vi "tearDown.vi"(8 "error in (no error)":errorcluster, 11 "reference in":refnum<class "Instrument Addon Scripting API Channels Unit Tests.lvclass">) -> (0 "error out":errorcluster, 3 "reference out":refnum<class "Instrument Addon Scripting API Channels Unit Tests.lvclass">)   [LabVIEW 2018, in "Instrument Addon Scripting API Channels Unit Tests.lvclass"]
doc: "tearDown runs after the test method has completed. Use this method to clean up any operations or references that were opened by setUp or the test method. Unit tests should be independent of other unit tests so this VI should ensure that the next test can run in a 'clean' test environment."
uses:
  Instrument Addon Scripting API Channels Unit Tests.lvclass
  Instrument Addon Scripting API Channels Unit Tests.lvclass/Instrument Addon Scripting API Channels Unit Tests.ctl
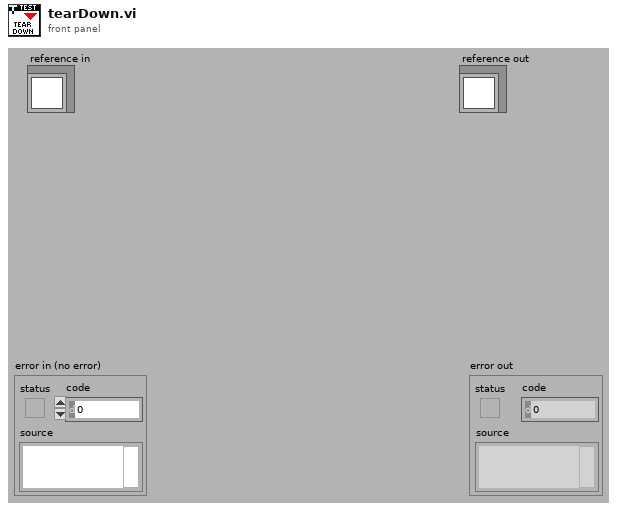
[diagram p1: front panel]
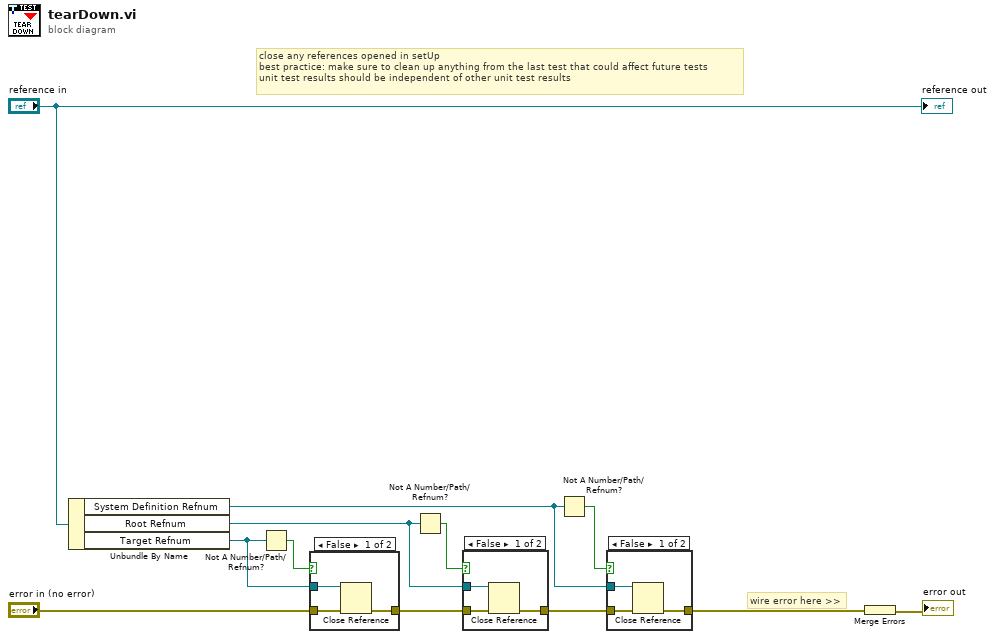
[diagram p0: block diagram]
diagram:
  # "wire error here >>"
  # "close any references opened in setUp\nbest practice: make sure to clean up anything from the last test that could affect future tests\nunit test results should be independent of other unit test results"
  n1 = Unbundle By Name("reference in") -> ("System Definition Refnum"=w3:refnum<k24>, "Root Refnum"=w5:refnum<k24>, "Target Refnum"=w7:refnum<k24>)
  n2 = Not A Number/Path/Refnum?(number/path/refnum=w7) -> (NaN/Path/Refnum?=w10:bool)
  n3 = case shown="False" w10 {
    tunnel: "error in (no error)" -> [w15 w16]
    tunnel: [w14 w16] -> w8
    tunnel: w7 -> [w13 _]
    frame False {
      n4 = Close Reference(reference=w13, error in (no error)=w15) -> (error out=w14:errorcluster)
    }
    frame True {
    }
  }
  n5 = Not A Number/Path/Refnum?(number/path/refnum=w5) -> (NaN/Path/Refnum?=w6:bool)
  n6 = case shown="False" w6 {
    tunnel: w8 -> [w19 w20]
    tunnel: w5 -> [w18 _]
    tunnel: [w17 w20] -> w2
    frame False {
      n7 = Close Reference(reference=w18, error in (no error)=w19) -> (error out=w17:errorcluster)
    }
    frame True {
    }
  }
  n8 = Not A Number/Path/Refnum?(number/path/refnum=w3) -> (NaN/Path/Refnum?=w4:bool)
  n9 = case shown="False" w4 {
    tunnel: w2 -> [w23 w24]
    tunnel: w3 -> [w22 _]
    tunnel: [w21 w24] -> w1
    frame False {
      n10 = Close Reference(reference=w22, error in (no error)=w23) -> (error out=w21:errorcluster)
    }
    frame True {
    }
  }
  n11 = Merge Errors(w1) -> (→"error out":errorcluster)
  "reference out" <- "reference in"
